vi "Read Network Interface.vi"(8 "error in (no error)":errorcluster, 11 "Transmission Data Unit in":refnum<class "Transmission Data Unit.lvclass">) -> (0 "error out":errorcluster, 2 "Network Interface":refnum<class "Network Interface.lvclass">, 3 "Transmission Data Unit out":refnum<class "Transmission Data Unit.lvclass">)   [LabVIEW 2021, in "Transmission Data Unit.lvclass"]
uses:
  Transmission Data Unit.lvclass
  Transmission Data Unit.lvclass/Transmission Data Unit.ctl
  Network Interface/Network Interface.lvclass
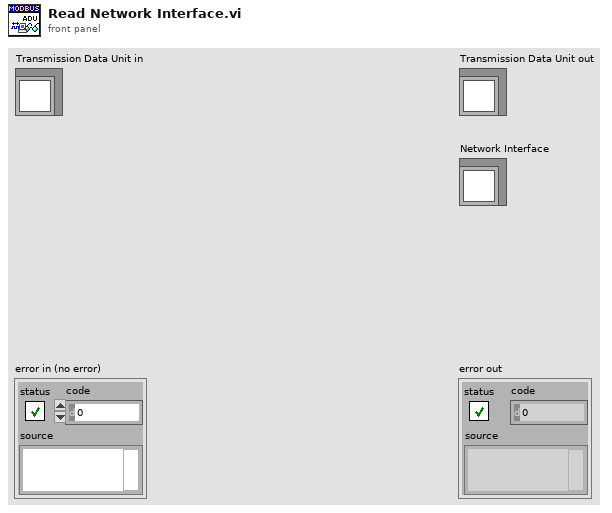
[diagram p1: front panel]
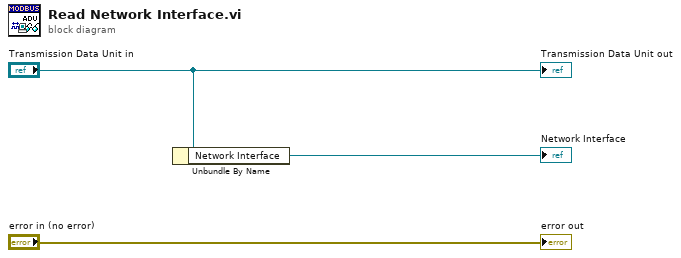
[diagram p0: block diagram]
diagram:
  n1 = Unbundle By Name("Transmission Data Unit in") -> ("Network Interface"=→"Network Interface":refnum<class "Network Interface.lvclass">)
  "error out" <- "error in (no error)"
  "Transmission Data Unit out" <- "Transmission Data Unit in"
